vi "GetHelp.vi"(11 "Restore in":refnum<class "Restore.lvclass">) -> (2 "Help":string, 3 "Restore out":refnum<class "Restore.lvclass">)   [LabVIEW 2014, in "Restore.lvclass"]
uses:
  Restore.lvclass
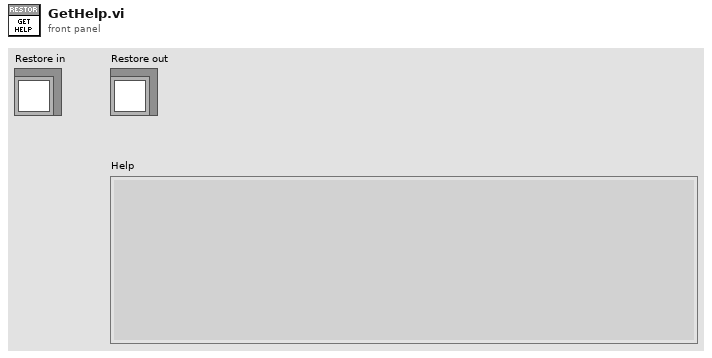
[diagram p1: front panel]
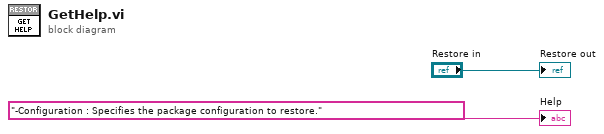
[diagram p0: block diagram]
diagram:
  "Restore out" <- "Restore in"
  "Help" <- "-Configuration : Specifies the package configuration to restore." ("Help")
